vi "ValidateInput.vi"(8 "error in (no error)":errorcluster, 10 "Input":string, 11 "BarCode in":refnum<class "BarCode.lvclass">) -> (0 "error out":errorcluster, 2 "OK":bool=TRUE, 3 "BarCode out":refnum<class "BarCode.lvclass">)   [LabVIEW 2013, in "BarCodes.lvlib" / "BarCode.lvclass"]
doc: "Returns whether the specified input can be expressed in this barcode format."
uses:
  BarCode.lvclass
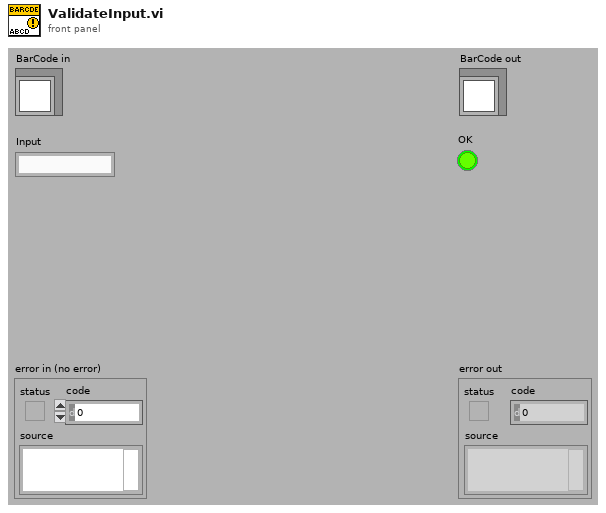
[diagram p1: front panel]
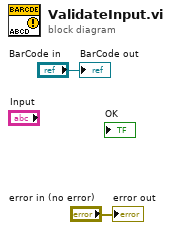
[diagram p0: block diagram]
diagram:
  "error out" <- "error in (no error)"
  "BarCode out" <- "BarCode in"
